vi "Untitled 1.vi"() -> ()   [LabVIEW 2019]
uses:
  <vilib>/addons/_NISVFA/_Shared subVIs/Common/SV Histogram from Buffered Data (1 Ch) (DBL).vi
  <vilib>/addons/_NISVFA/_Shared subVIs/Common/svc_Increment Histogram and Count.vi
  <vilib>/addons/_NISVFA/_Shared subVIs/Common/svc_Value to Histogram Bin Index.vi
  <vilib>/addons/_NISVFA/_Shared subVIs/Common/svc_Generate Bins from Range and Intervals.vi
  <vilib>/addons/_NISVFA/_Shared subVIs/Common/svc_Input Array to Histogram Bin Configuration.vi
  <vilib>/Analysis/NI_AALPro.lvlib
panel:
  out "error":i32
  out "# outside":cluster{"total":i32, "below":i32, "above":i32}
  out "Axis":dbl[](array[numeric]) format="%0.2f"
  out "Histogram":i32[](array[numeric])
  out "Histogram Graph":T1(graph)
  in  "inclusion":enum32{"lower", "upper"}(ring)
  in  "# bins":i32
  in  "min":dbl format="%0.2f"
  in  "max":dbl format="%0.2f"
  in  "Bins":T2(array[cluster]) {"upper" format="%0.2f"; "lower" format="%0.2f"}
  out "actual range":cluster{"minimum":dbl, "maximum":dbl}={"minimum"=-10.0, "maximum"=10.0}
  out "histogram":cluster{"bin centers":dbl[], "counts":u64[]}(graph)
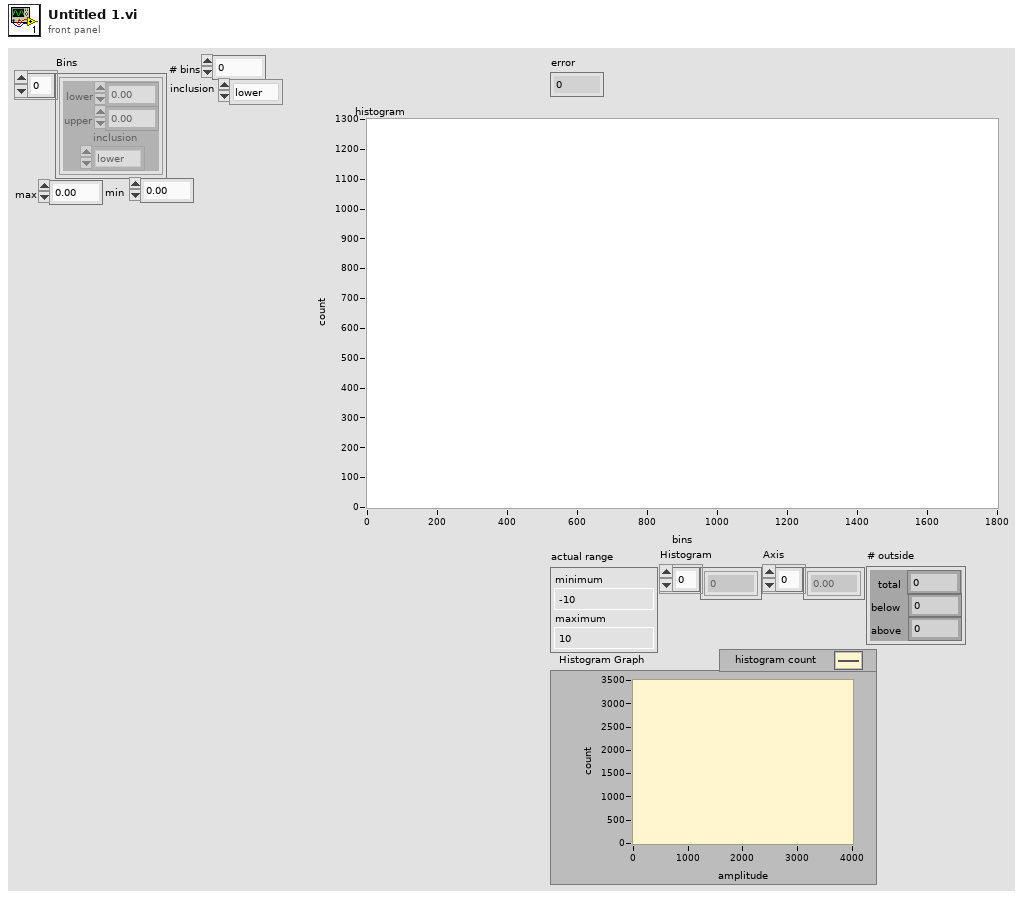
[diagram p1: front panel]
types:
  T1 = cluster{"X Values":dbl[], "Histogram: h(x)":i32[]}
  T2 = cluster{"lower":dbl, "upper":dbl, "inclusion":enum32{"lower", "upper", "both", "neither"}}[]
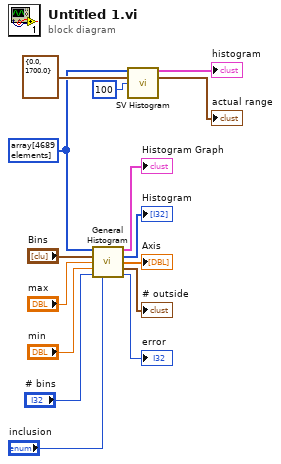
[diagram p0: block diagram]
diagram:
  w11 = u32[] array[4689 elements] ("number")
  n1 = call <vilib>:"General Histogram.vi"("X"=w11, "Bins"="Bins", "max"="max", "min"="min", "# bins"="# bins", "inclusion"="inclusion") -> ("Histogram Graph"=→"Histogram Graph":T1, "Histogram"=→"Histogram":i32[], "Axis"=→"Axis":dbl[], "# outside"=→"# outside":cluster{"total":i32, "below":i32, "above":i32}, "error"=→"error":i32)  [unwired: 5 in]
  n2 = call-poly <vilib>:"SV Histogram.vi"("new data"=w11, "range"=cluster{"minimum":dbl, "maximum":dbl} {"minimum"=0.0, "maximum"=1700.0}, "number of bins (20)"=100) -> ("histogram"=→"histogram":cluster{"bin centers":dbl[], "counts":u64[]}, "actual range"=→"actual range":cluster{"minimum":dbl, "maximum":dbl})  [unwired: 10 in, 1 out]
